vi "Output Impedance Test.vi"(0 "TSM context":T1, 5 "Capture Time (s)":dbl=0.005 format="%#_13g") -> (15 "error out":errorcluster)   [LabVIEW 2020]
doc: "VI determines the ouput impedence of the DUT by measuring voltage differences on No Load and Loaded conditions using a external resistance circuitary."
uses:
  <vilib>/NI_TestStand_SemiconductorModule/NI_TestStand_Semiconductor_Module.lvlibp/PinMap/General/SemiconductorModuleContext.ctl
  242b611e-b79a-40ea-b4d4-c5563d0fb6c2.vi
  f7f5d33f-d09a-4d82-ae73-b91c36f905d8.vi
  a6faa0e4-c21c-4b44-add0-1e29a5c14142.vi
  242b611e-b79a-40ea-b4d4-c5563d0fb6c2.vi/f50271b6-cec7-411a-9124-7216d9482ac8.vi
  <vilib>/NI_TestStand_SemiconductorModule/NI_TestStand_Semiconductor_Module.lvlibp/PinMap/Relay Driver/ControlRelay(s).vi
  <vilib>/NI_TestStand_SemiconductorModule/NI_TestStand_Semiconductor_Module.lvlibp/PinMap/Relay Driver/ApplyRelayConfiguration.vi
  <vilib>/Utility/High Resolution Polling Wait.vi
  <vilib>/measure/matone.llb/Extract Single Tone Information N Chan.vi
  <vilib>/NI_TestStand_SemiconductorModule/NI_TestStand_Semiconductor_Module.lvlibp/PinMap/General/Publish/PublishDataDoubleFunctionalTest.vi
  <vilib>/NI_TestStand_SemiconductorModule/NI_TestStand_Semiconductor_Module.lvlibp
  <vilib>/measure/NI_MAPro.lvlib
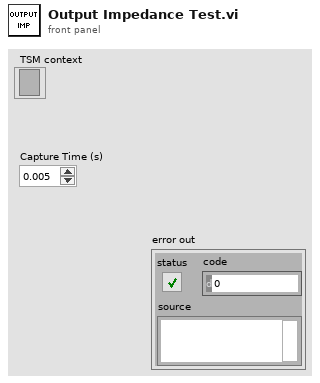
[diagram p1: front panel]
types:
  T1 = typedef "NI_TestStand_Semiconductor_Module.lvlibp/SemiconductorModuleContext.ctl" = refnum<k7>
  T2 = cluster{"approx freq. (optional)":dbl, "search (+/- % of Fsampl.)":dbl}
  T3 = typedef "TSM DAQmx Multi-Task.ctl" = cluster{"Pin Query Context":refnum<class "MultiplePinMultipleSessionQueryContext.lvclass">, "SSC":T4[], "Site Numbers":i32[], "Pins":tag[]}
  T4 = typedef "SSC DAQmx.ctl" = cluster{"DAQmx Task ":refnum<k21>, "Channels":string, "Channel Lists":string}
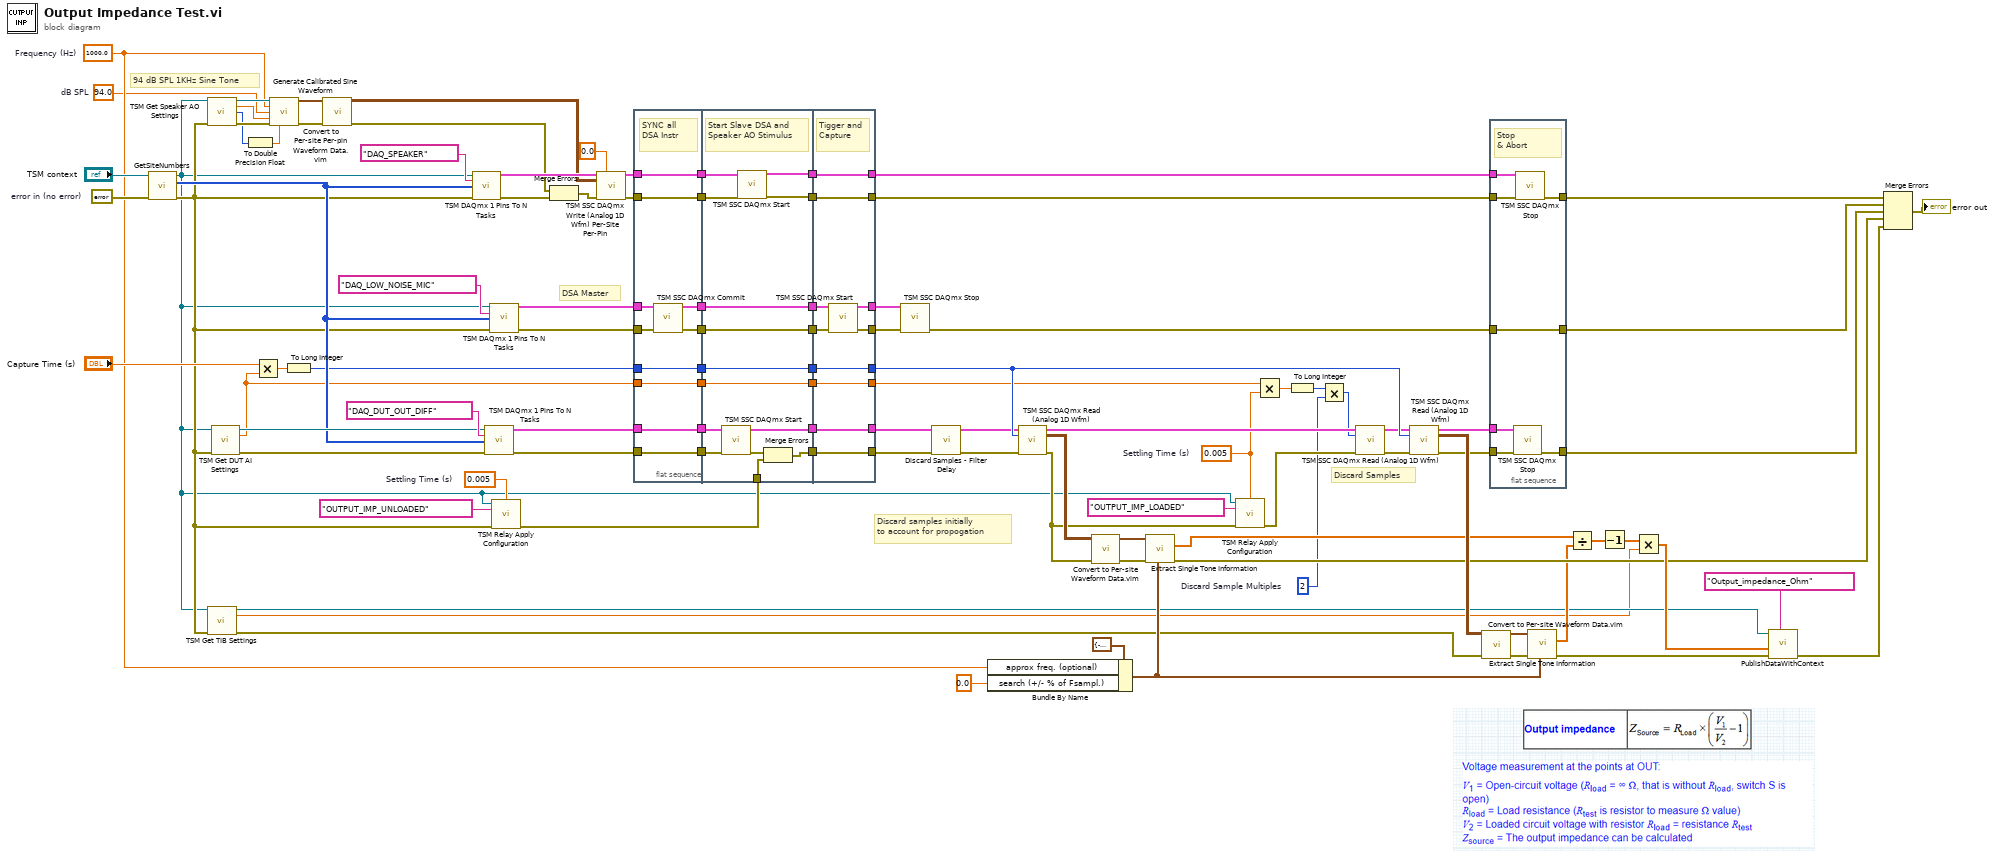
[diagram p0: block diagram]
diagram:
  w25 = 2  # Discard Sample Multiples
  w5 = 94.0  # dB SPL
  w6 = 1000.0  # Frequency (Hz)
  w86 = 0.005  # Settling Time (s)
  w28 = 0.005  # Settling Time (s)
  w94 = errorcluster {"status"=FALSE, "code"=0, "source"=""}  # error in (no error)
  # "Discard samples initially\nto account for propogation"
  # "Discard Samples"
  # "DSA Master"
  # "94 dB SPL 1KHz Sine Tone"
  n1 = call <vilib>:"GetSiteNumbers.vi"("error in (no error)"=w94, "Semiconductor Module Context"="TSM context") -> ("error out"=w13:errorcluster, "Site Numbers"=w61:i32[], "Semiconductor Module Context Out"=w10:T1)  [unwired: 6 in, 1 out]
  n2 = call "TSM Get Speaker AO Settings.vi"("TSM context"=w10, "error in (no error)"=w13) -> ("TSM context Out"=w7:T1, "Sampling Rate (Hz)"=w4:dbl, "Samples per channel"=w2:i32, "error out"=w9:errorcluster)  [unwired: 9 in, 1 out]
  n3 = call "TSM Get TIB Settings.vi"("TSM context In"=w10, "error in (no error)"=w13) -> ("TSM context Out"=w67:T1, "External Resistance (Ohm)"=w65:dbl, "error out"=w17:errorcluster)  [unwired: 11 in]
  n4 = call "TSM Get DUT AI Settings.vi"("TSM context"=w10, "error in (no error)"=w13) -> ("TSM context Out"=w92:T1, "Sampling Rate (Hz)"=w35:dbl, "error out"=w66:errorcluster)  [unwired: 9 in, 2 out]
  n5 = To Double Precision Float(number=w2) -> (double precision float=w1:dbl)
  n6 = Multiply(x="Capture Time (s)", y=w35) -> (x*y=w37:dbl)
  n7 = call "Generate Calibrated Sine Waveform.vi"("TSM context"=w7, "Frequency (Hz)"=w6, "dB SPL"=w5, "Sampling Rate (Hz)"=w4, "error in (no error)"=w9, "Samples per channel"=w1) -> ("Per-Site Waveforms Out"=w3:waveform(dbl)[], "error out"=w8:errorcluster)  [unwired: 7 in, 1 out]
  n8 = To Long Integer(number=w37) -> (32bit integer=w36:i32)
  n9 = call "Convert to Per-site Per-pin Waveform Data.vim"("Waveform In"=w3) -> ("Per Site Per Pin Waveform Out"=w63:waveform(dbl)[][])  [unwired: 14 in]
  n10 = call "TSM DAQmx 1 Pins To N Tasks.vi"("TSM context"=w10, "Pins"=tag "DAQ_SPEAKER", "Site Numbers"=w61, "error in"=w13) -> ("DAQ TSM Out"=w79:T3, "error out"=w64:errorcluster)  [unwired: 10 in]
  n11 = call "TSM DAQmx 1 Pins To N Tasks.vi"("TSM context"=w92, "Pins"=tag "DAQ_DUT_OUT_DIFF", "Site Numbers"=w61, "error in"=w66) -> ("DAQ TSM Out"=w91:T3, "error out"=w15:errorcluster)  [unwired: 10 in]
  n12 = call "TSM DAQmx 1 Pins To N Tasks.vi"("TSM context"=w10, "Pins"=tag "DAQ_LOW_NOISE_MIC", "Site Numbers"=w61, "error in"=w13) -> ("DAQ TSM Out"=w49:T3, "error out"=w50:errorcluster)  [unwired: 10 in]
  n13 = call "TSM Relay Apply Configuration.vi"("TSM Context"=w10, "Settling Time (0s)"=w86, "Relay Configuration"=tag "OUTPUT_IMP_UNLOADED", "error in (no error)"=w13) -> ("error out"=w14:errorcluster)  [unwired: 11 in]
  n14 = Merge Errors(w8, w64) -> (w12:errorcluster)
  n15 = call "TSM SSC DAQmx Write (Analog 1D Wfm) Per-Site Per-Pin.vi"("DAQ TSM in"=w79, "Idle Channel Value (0)"=0.0, "Per-Site Per-Pin Waveforms in"=w63, "error in"=w12) -> ("DAQ TSM Out"=w43:T3, "error out"=w44:errorcluster)  [unwired: 10 in]
  n16 = flat-sequence {
    tunnel: w36 -> [w106]
    tunnel: w43 -> [w107]
    tunnel: w44 -> [w108]
    tunnel: w91 -> [w109]
    tunnel: w15 -> [w110]
    tunnel: [w110] -> w55
    tunnel: [w109] -> w54
    tunnel: [w108] -> w53
    tunnel: [w107] -> w52
    tunnel: [w106] -> w51
    tunnel: w50 -> [w105]
    tunnel: w49 -> [w104]
    tunnel: [w103] -> w48
    tunnel: [w102] -> w46
    tunnel: w35 -> [w101]
    tunnel: [w101] -> w33
    tunnel: [w112] -> w60
    tunnel: [w119] -> w59
    tunnel: [w117] -> w58
    tunnel: [w114] -> w57
    tunnel: [w124] -> w56
    tunnel: w55 -> [w121]
    tunnel: w54 -> [w120]
    tunnel: w53 -> [w115]
    tunnel: w52 -> [w116]
    tunnel: w51 -> [w124]
    tunnel: w48 -> [w122]
    tunnel: [w123] -> w47
    tunnel: w46 -> [w123]
    tunnel: [w122] -> w45
    tunnel: [w113] -> w34
    tunnel: w33 -> [w113]
    tunnel: w14 -> [w111]
    tunnel: [w132] -> w98
    tunnel: [w133] -> w99
    tunnel: [w130] -> w22
    tunnel: [w131] -> w19
    tunnel: [w134] -> w88
    tunnel: w60 -> [w130]
    tunnel: w59 -> [w131]
    tunnel: w58 -> [w132]
    tunnel: w57 -> [w133]
    tunnel: w56 -> [w134]
    tunnel: w47 -> [w128]
    tunnel: w45 -> [w129]
    tunnel: [w127] -> w42
    tunnel: [w126] -> w41
    tunnel: [w125] -> w20
    tunnel: w34 -> [w125]
    frame #0 {
      # "SYNC all DSA Instr"
      n17 = call "TSM SSC DAQmx Commit.vi"("TSM DAQmx In"=w104, "error in (no error)"=w105) -> ("TSM DAQmx Out"=w102:T3, "error out"=w103:errorcluster)  [unwired: 12 in]
    }
    frame #1 {
      # "Start Slave DSA and Speaker AO Stimulus"
      n18 = call "TSM SSC DAQmx Start.vi"("TSM DAQmx In"=w120, "error in (no error)"=w121) -> ("TSM DAQmx Out"=w119:T3, "error out"=w118:errorcluster)  [unwired: 12 in]
      n19 = call "TSM SSC DAQmx Start.vi"("TSM DAQmx In"=w116, "error in (no error)"=w115) -> ("TSM DAQmx Out"=w114:T3, "error out"=w117:errorcluster)  [unwired: 12 in]
      n20 = Merge Errors(w118, w111) -> (w112:errorcluster)
    }
    frame #2 {
      # "Tigger and Capture"
      n21 = call "TSM SSC DAQmx Start.vi"("TSM DAQmx In"=w128, "error in (no error)"=w129) -> ("TSM DAQmx Out"=w126:T3, "error out"=w127:errorcluster)  [unwired: 12 in]
    }
  }
  n22 = call "TSM SSC DAQmx Stop.vi"("TSM DAQmx In"=w41, "error in (no error)"=w42) -> ("error out"=w40:errorcluster)  [unwired: 12 in, 1 out]
  n23 = call "Discard Samples - Filter Delay.vi"("DAQ TSM in"=w19, "error in"=w22) -> ("DAQ TSM Out"=w18:T3, "error out"=w21:errorcluster)  [unwired: 12 in]
  n24 = Bundle By Name(cluster=T2 {"approx freq. (optional)"=-1.0, "search (+/- % of Fsampl.)"=5.0} ("advanced search"), "approx freq. (optional)"=w6, "search (+/- % of Fsampl.)"=0.0) -> (w69:T2)
  n25 = call "TSM SSC DAQmx Read (Analog 1D Wfm).vi"("DAQ TSM in"=w18, "Samples to read"=w88, "error in"=w21) -> ("DAQ TSM Out"=w31:T3, "Per-Site Per-Pin Waveforms Out"=w97:waveform(dbl)[][], "error out"=w77:errorcluster)  [unwired: 10 in]
  n26 = call "Convert to Per-site Waveform Data.vim"("Per-Site Per-Pin Waveform In"=w97) -> ("Per-Site Waveform Out"=w76:waveform(dbl)[])  [unwired: 14 in]
  n27 = call-poly <vilib>:"Extract Single Tone Information.vi"("advanced search"=w69, "error in (no error)"=w77, "time signals in"=w76) -> ("error out"=w75:errorcluster, "detected amplitudes"=w74:dbl[])  [unwired: 3 in, 4 out]
  n28 = call "TSM Relay Apply Configuration.vi"("TSM Context"=w10, "Settling Time (0s)"=w28, "Relay Configuration"=tag "OUTPUT_IMP_LOADED", "error in (no error)"=w77) -> ("error out"=w32:errorcluster)  [unwired: 11 in]
  n29 = Multiply(x=w20, y=w28) -> (x*y=w27:dbl)
  n30 = To Long Integer(number=w27) -> (32bit integer=w26:i32)
  n31 = Multiply(x=w26, y=w25) -> (x*y=w24:i32)
  n32 = call "TSM SSC DAQmx Read (Analog 1D Wfm).vi"("DAQ TSM in"=w31, "Samples to read"=w24, "error in"=w32) -> ("DAQ TSM Out"=w30:T3, "error out"=w29:errorcluster)  [unwired: 10 in, 1 out]
  n33 = call "TSM SSC DAQmx Read (Analog 1D Wfm).vi"("DAQ TSM in"=w30, "Samples to read"=w88, "error in"=w29) -> ("DAQ TSM Out"=w87:T3, "Per-Site Per-Pin Waveforms Out"=w85:waveform(dbl)[][], "error out"=w16:errorcluster)  [unwired: 10 in]
  n34 = call "Convert to Per-site Waveform Data.vim"("Per-Site Per-Pin Waveform In"=w85) -> ("Per-Site Waveform Out"=w71:waveform(dbl)[])  [unwired: 14 in]
  n35 = flat-sequence {
    tunnel: w99 -> [w137]
    tunnel: w98 -> [w138]
    tunnel: w87 -> [w141]
    tunnel: w16 -> [w140]
    tunnel: [w139] -> w11
    tunnel: [w136] -> w96
    tunnel: w40 -> [w135]
    tunnel: [w135] -> w39
    frame #0 {
      # "Stop \n& Abort"
      n36 = call "TSM SSC DAQmx Stop.vi"("TSM DAQmx In"=w141, "error in (no error)"=w140) -> ("error out"=w139:errorcluster)  [unwired: 12 in, 1 out]
      n37 = call "TSM SSC DAQmx Stop.vi"("TSM DAQmx In"=w137, "error in (no error)"=w138) -> ("error out"=w136:errorcluster)  [unwired: 12 in, 1 out]
    }
  }
  n38 = call-poly <vilib>:"Extract Single Tone Information.vi"("advanced search"=w69, "error in (no error)"=w17, "time signals in"=w71) -> ("error out"=w68:errorcluster, "detected amplitudes"=w70:dbl[])  [unwired: 3 in, 4 out]
  n39 = Divide(x=w74, y=w70) -> (x/y=w84:dbl[])
  n40 = Decrement(x=w84) -> (x-1=w83:dbl[])
  n41 = Multiply(x=w83, y=w65) -> (x*y=w82:dbl[])
  n42 = call-poly <vilib>:"PublishDataWithContext.vi"("Published Data Id"=tag "Output_impedance_Ohm", "error in (no error)"=w68, "Data In"=w82, "Semiconductor Module Context"=w67) -> ("error out"=w81:errorcluster)  [unwired: 6 in, 1 out]
  n43 = Merge Errors(w96, w39, w11, w75, w81) -> (→"error out":errorcluster)
